vi "Send GUID to Server Listener.vi"(8 "error in (no error)":errorcluster, 11 "Client Controller in":refnum<class "Client Controller.lvclass">) -> (0 "error out":errorcluster, 3 "Client Controller out":refnum<class "Client Controller.lvclass">)   [LabVIEW 2013, in "Client Controller.lvlib" / "Client Controller.lvclass"]
uses:
  Client Controller.lvclass
  Client Controller.lvclass/Client Controller.ctl
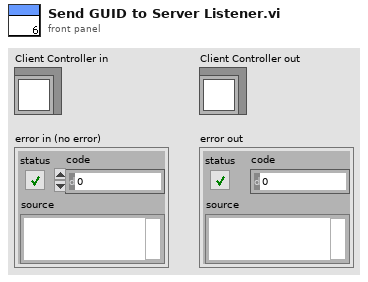
[diagram p1: front panel]
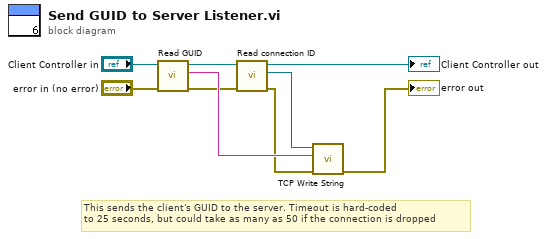
[diagram p0: block diagram]
diagram:
  # "This sends the client's GUID to the server. Timeout is hard-coded\nto 25 seconds, but could take as many as 50 if the connection is dropped"
  n1 = call "Read GUID.vi"("error in (no error)"="error in (no error)", "Client Controller in"="Client Controller in") -> ("error out"=w2:errorcluster, "GUID"=w6:string, "Client Controller out"=w5:refnum<class "Client Controller.lvclass">)  [unwired: 7 in]
  n2 = call "Read connection ID.vi"("error in (no error)"=w2, "Client Controller in"=w5) -> ("error out"=w1:errorcluster, "connection ID"=w3:refnum<k5>, "Client Controller out"=→"Client Controller out":refnum<class "Client Controller.lvclass">)  [unwired: 7 in]
  n3 = call <vilib>:"TCP Write String.vi"("error in (no error)"=w1, "data in"=w6, "connection ID"=w3) -> ("error out"=→"error out":errorcluster)  [unwired: 7 in, 1 out]
